vi "Grouped Interface.vi"() -> ()   [LabVIEW 2020, in "Grouped Interface.lvlib"]
doc: "This template is based off of the Queued Message Handler design pattern and the Queued Message Handler project template that ships with LabVIEW.\n\nThe main difference is that the queue is private to this module and communication between modules is performed via Broadcast and Request events.\n\nRequest events are wrapped in public API methods and are handled in the Event Handling Loop (EHL) of this VI. Any module can register for Broadcast events sent by this module. The EHL generates messages based on user interface actions.\n\nThe Message Handling Loop (MHL) processes messages generated by the EHL, or by other messages. The messages are string values, so new messages can be added easily to the Message Cases case structure in the MHL. Each message cluster can also provide an optional value for Message Data, which is a variant that can be converted to whatever message-specific data is required.\n_____\nBased on DQMH Project Template 7.0.1.1316."
uses:
  Grouped Interface.lvlib
  Grouped Interface/User Data--cluster.ctl
  <vilib>/Utility/miscctls.llb/LVRectTypeDef.ctl
  <vilib>/Utility/miscctls.llb/LVPointTypeDef.ctl
  Grouped Interface/Window Size Change Arguments--cluster.ctl
  Grouped Interface/Item Selected Arguments--cluster.ctl
  b692cfee-ccc7-4fcf-b071-59a242409c2d.vi
  6dcf879b-e50e-4c79-86d4-cf94ad6efafd.vi
  83f7a507-39ed-4955-bda1-3ff58afc1cf6.vi
  e3bdbc03-a268-4972-8073-54fcde4bb4c7.vi
  aefe27f5-81e8-4736-98ba-c14e2c182a52.vi
  b14c7c30-2e35-4566-a836-13db9432b85a.vi
  <userlib>/_NEVSTOP/Communicable State Machine(CSM)/AdvanceAPI/CSM - Revert Arguments-Safe String.vi
  <userlib>/_NEVSTOP/Communicable State Machine(CSM)/_Shared/Trim Single-line Text.vi
  <userlib>/_NEVSTOP/Communicable State Machine(CSM)/AdvanceAPI/CSM - Make String Arguments Safe.vi
  <userlib>/_NEVSTOP/Communicable State Machine(CSM)/AdvanceAPI/CSM - Break Down Multiple States String.vi
  <userlib>/_NEVSTOP/Communicable State Machine(CSM)/AdvanceAPI/CSM - Compact Multiple States.vi
  <userlib>/_NEVSTOP/Communicable State Machine(CSM)/AdvanceAPI/CSM - Keywords.vi
  <userlib>/_NEVSTOP/Communicable State Machine(CSM)/addons/API-String-Arugments-Support/_Support/Convert API String Arguments to Data(variant).vi
  <userlib>/_NEVSTOP/Communicable State Machine(CSM)/addons/API-String-Arugments-Support/_Support/Data To API String Arguments.vi
  <vilib>/Comparison/Equal/Equal Functor/Equal Functor.lvclass
  <userlib>/_NEVSTOP/Communicable State Machine(CSM)/Communicable State Machine.lvlib
panel:
  in  "min":bool
  in  "close":bool
  in  "Name (\"\" to Use UUID)":string="Main UI"
  out "State History":string
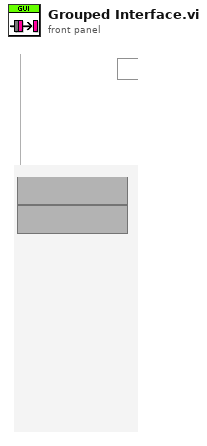
[diagram p1: front panel]
types:
  T1 = enum32{"Invalid", "Standard", "Closed", "Hidden", "Minimized", "Maximized"}
  T2 = enum32{"invalid app kind", "Development System", "Run Time System", "Student Edition", "Embedded LabVIEW", "Evaluation", "Custom"}
  T3 = typedef "Grouped Interface.lvlib/User Data--cluster.ctl" = cluster{"SubPanels":refnum<vi>[], "Interface Module List":string[], "Window Bounds":T4, "Function Module List":set{string}}
  T4 = typedef "LVRectTypeDef.ctl" = cluster{"Left":i16, "Top":i16, "Right":i16, "Bottom":i16}
  T5 = typedef "Grouped Interface.lvlib/Window Size Change Arguments--cluster.ctl" = cluster{"Module Name":string, "Window Size":T4}
  T6 = typedef "Grouped Interface.lvlib/Item Selected Arguments--cluster.ctl" = cluster{"Module Name":string, "Item Name":string}
  T7 = typedef "Communicable State Machine.lvlib/_CSM_Response Source Message.ctl" = cluster{"‘State":string, "’Arguments":string, "’Error":errorcluster}
  T8 = cluster{"Current VI Reference":refnum<vi>, "Close Panel on Exit?":bool}
  T9 = cluster{"Core":cluster{"Current VI Reference":refnum<vi>, "Close Panel on Exit?":bool}, "User Data":T3}
  T10 = typedef "LVPointTypeDef.ctl" = cluster{"Horizontal":i16, "Vertical":i16}
  T11 = typedef "Grouped Interface.lvlib/Module Definition--cluster.ctl" = cluster{"模块名称":string, "项定义":T12[]}
  T12 = typedef "Grouped Interface.lvlib/Function Item--cluster.ctl" = cluster{"项名":string, "符号图形路径":path}
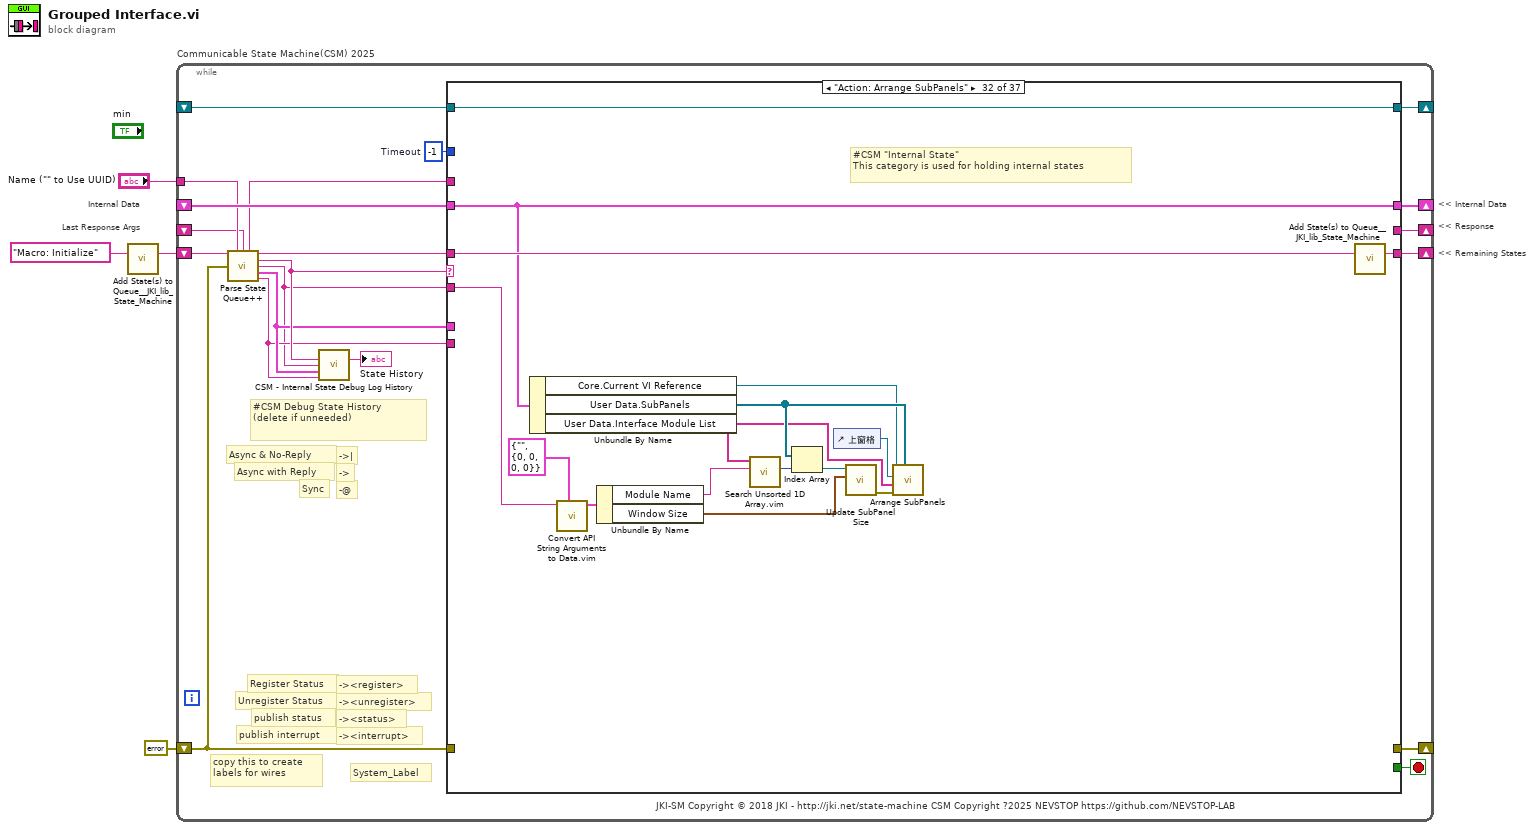
[diagram p0: block diagram]
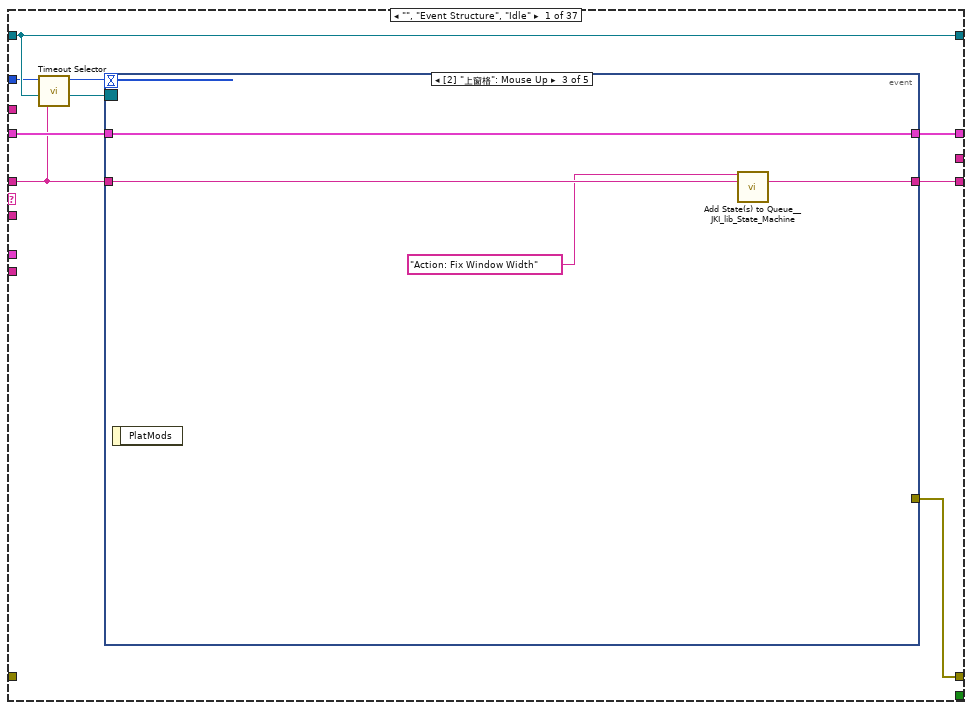
[diagram p2: hidden frame]
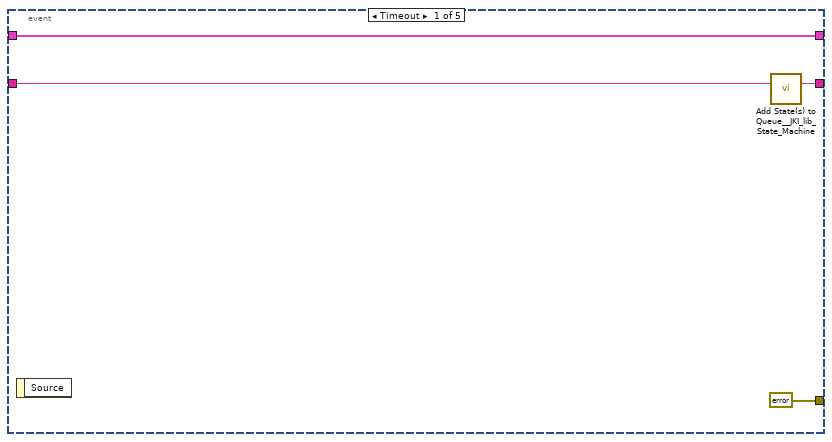
[diagram p3: hidden frame]
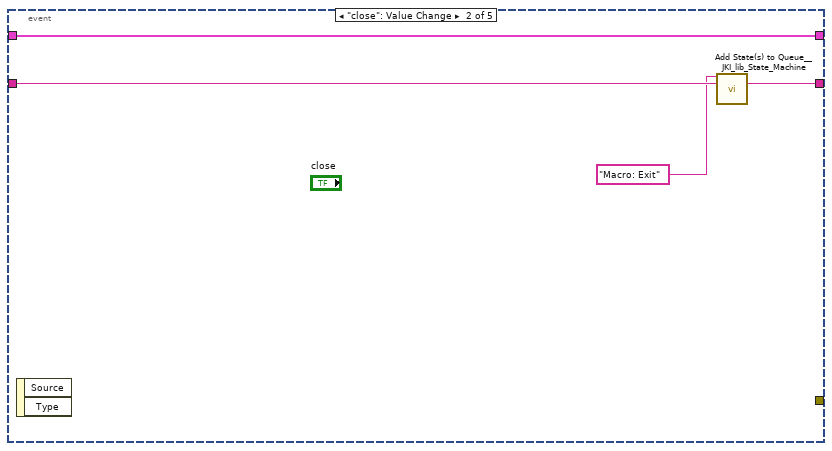
[diagram p4: hidden frame]
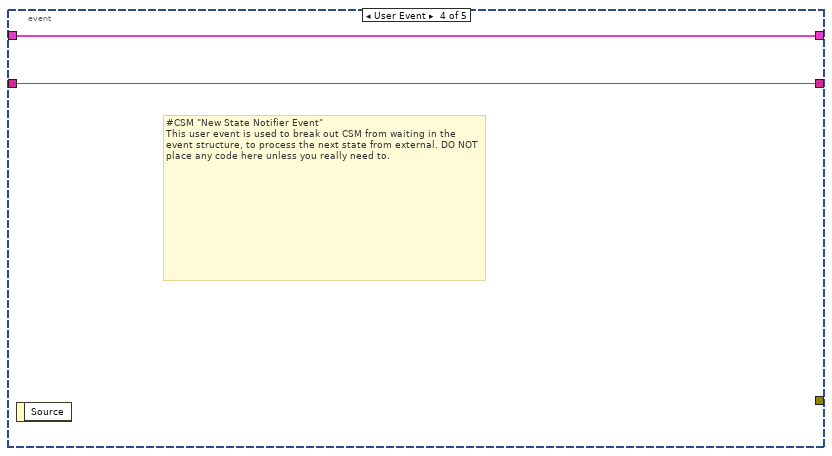
[diagram p5: hidden frame]
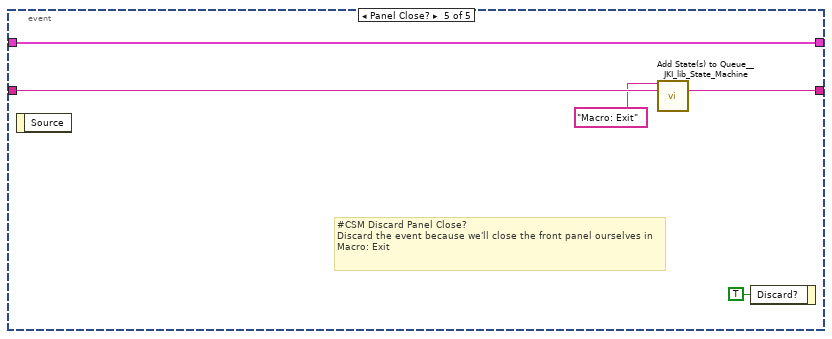
[diagram p6: hidden frame]
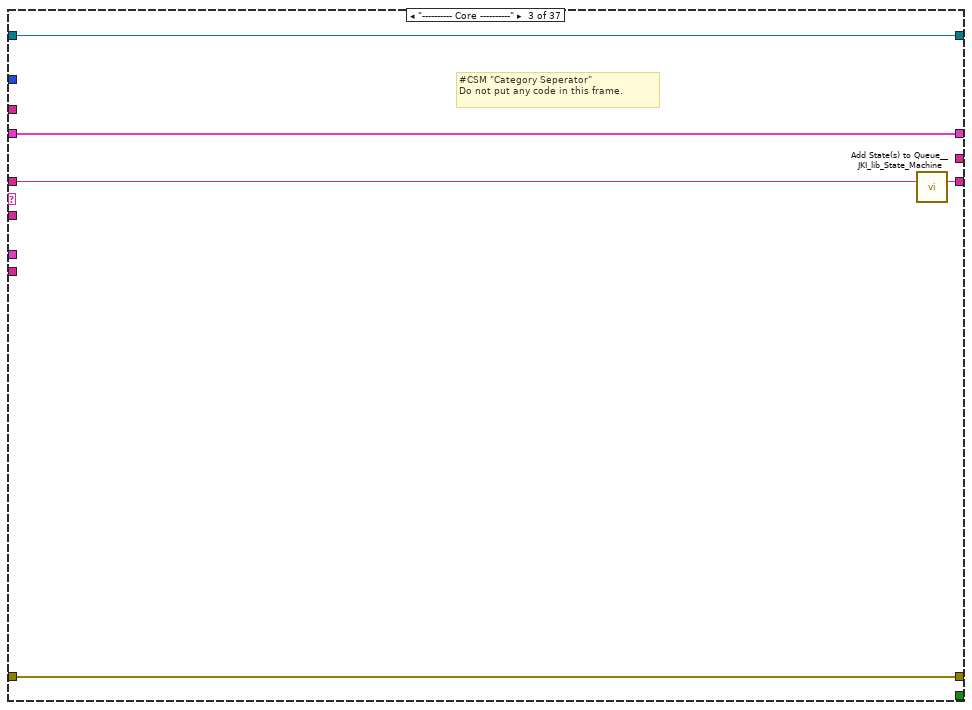
[diagram p8: hidden frame]
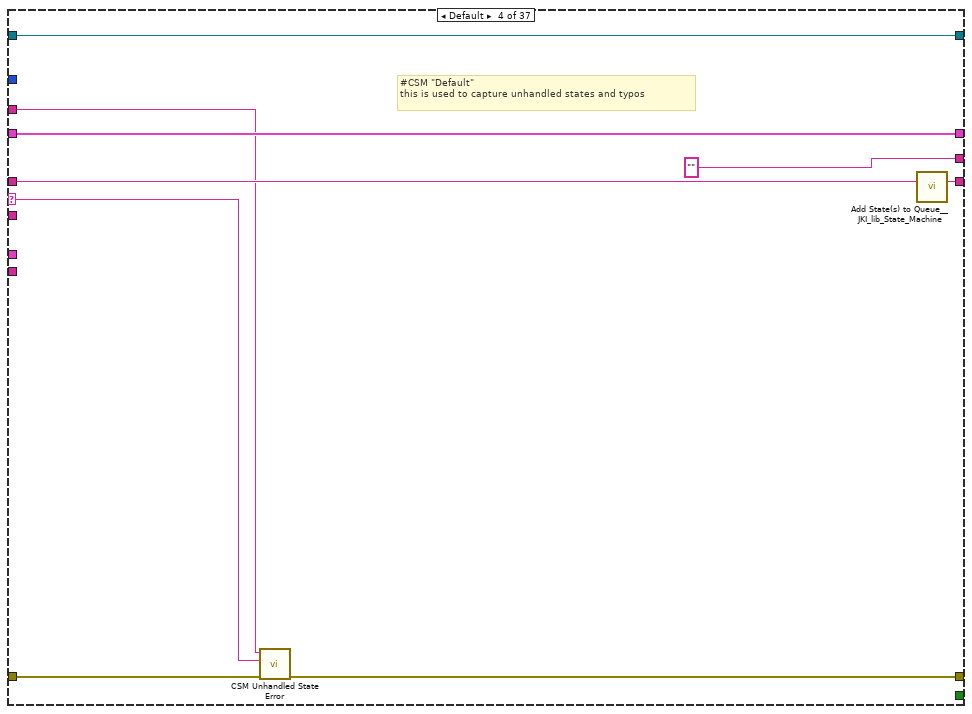
[diagram p9: hidden frame]
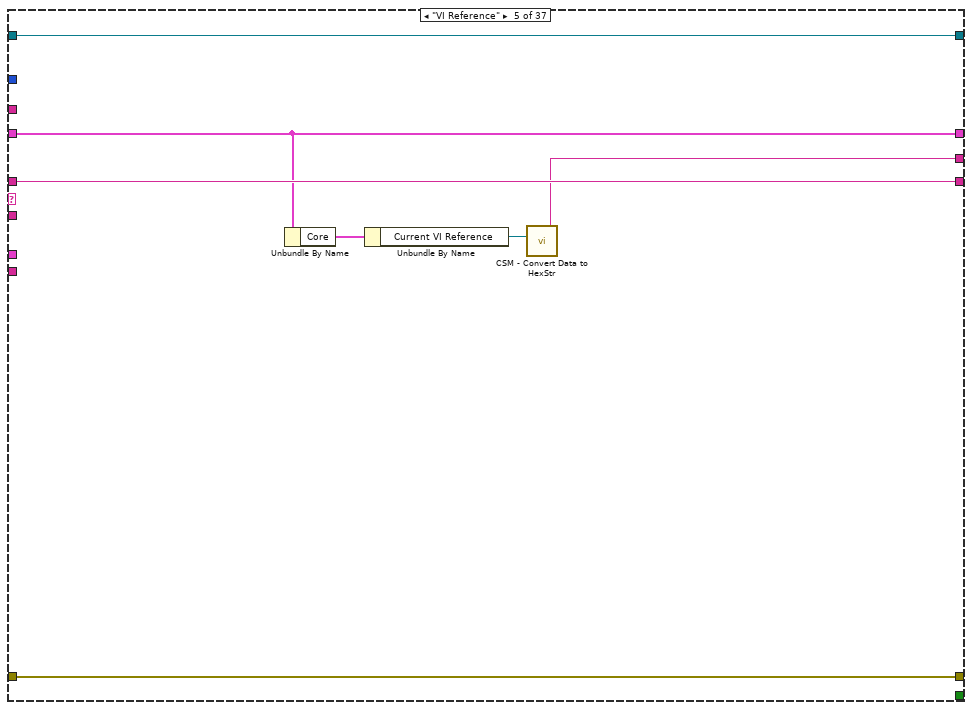
[diagram p10: hidden frame]
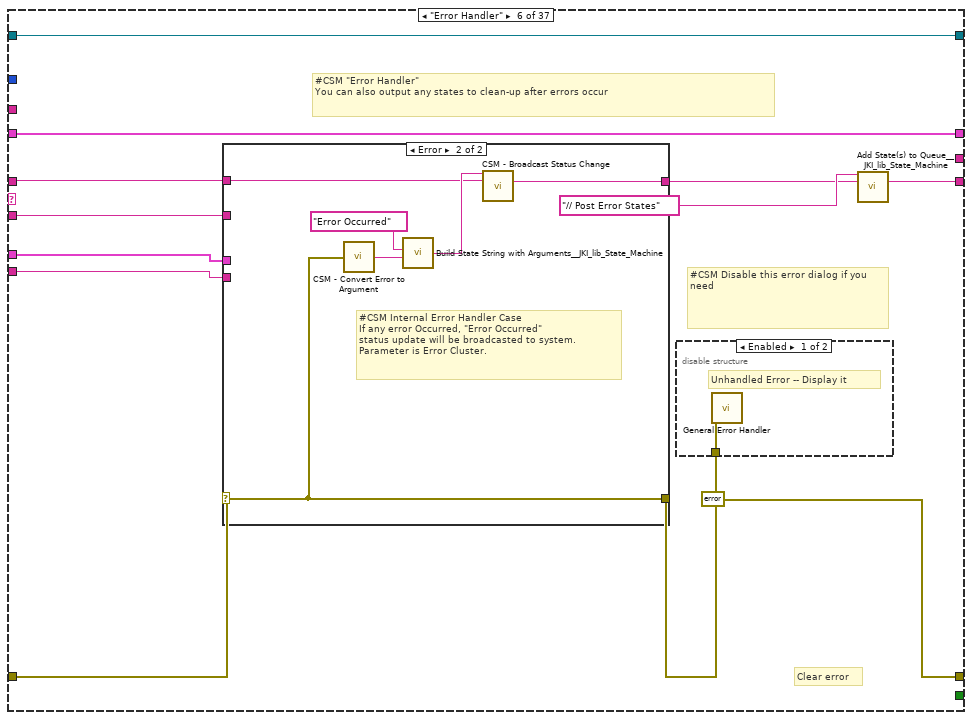
[diagram p11: hidden frame]
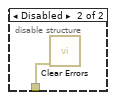
[diagram p12: hidden frame]
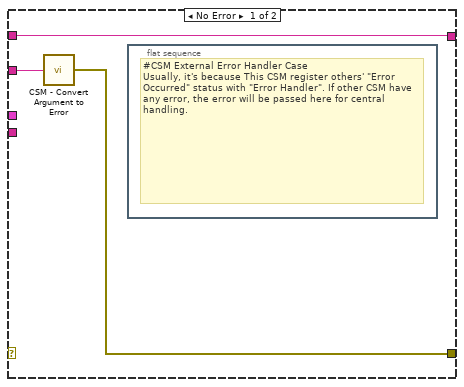
[diagram p13: hidden frame]
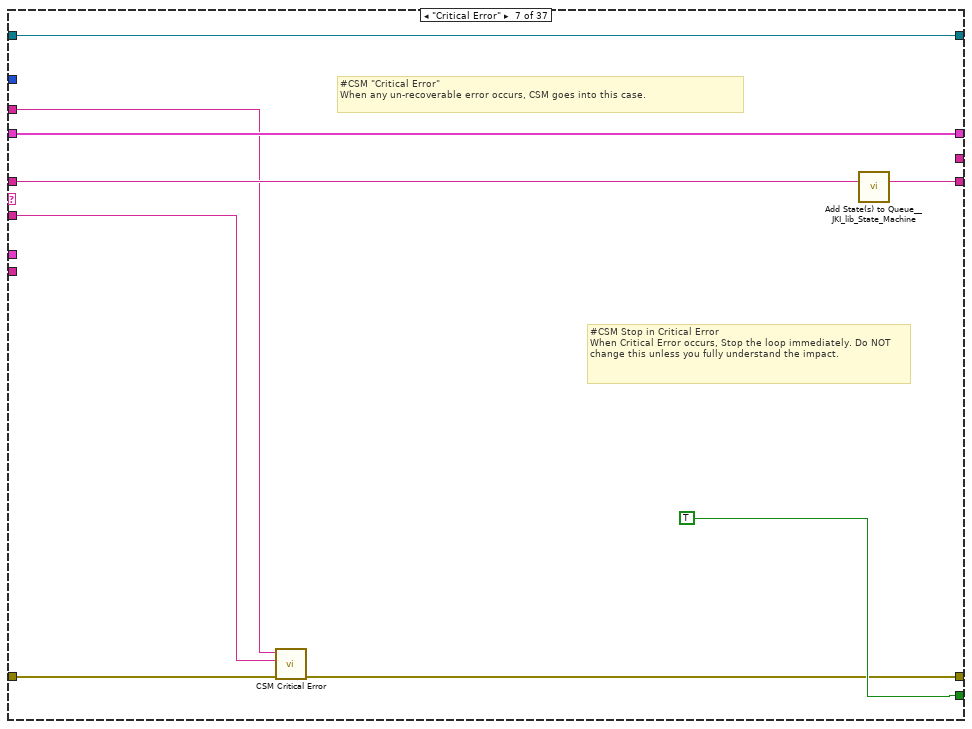
[diagram p14: hidden frame]
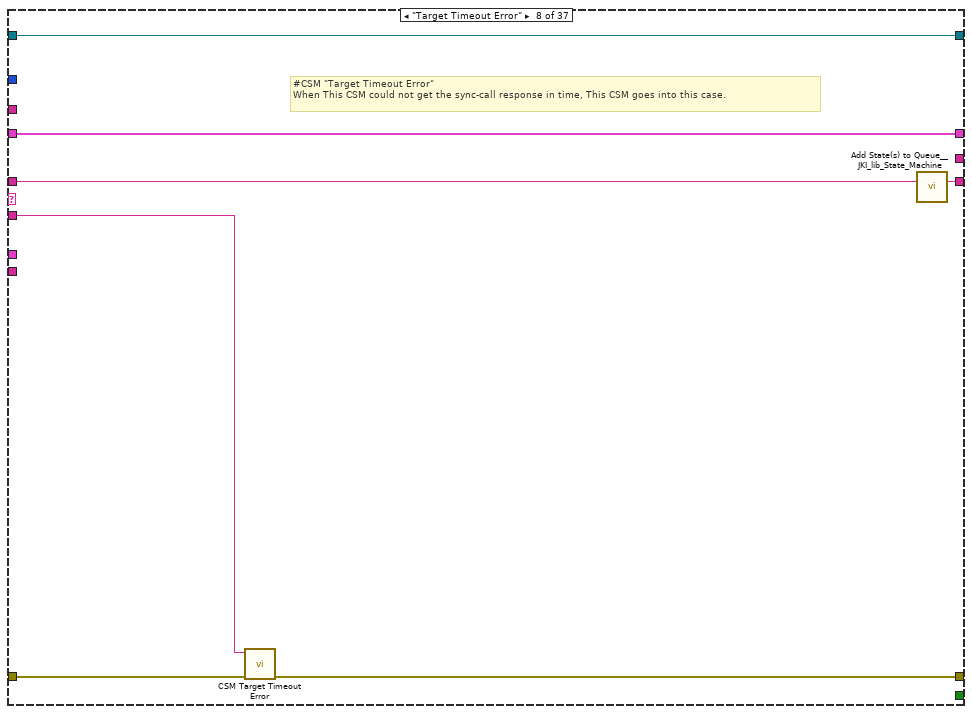
[diagram p15: hidden frame]
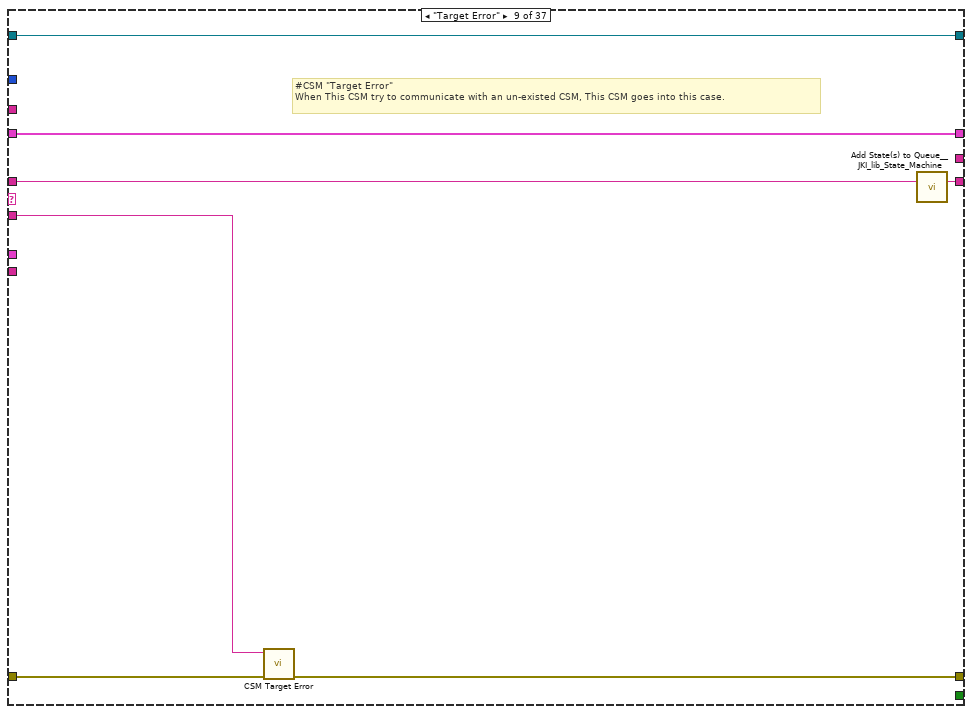
[diagram p16: hidden frame]
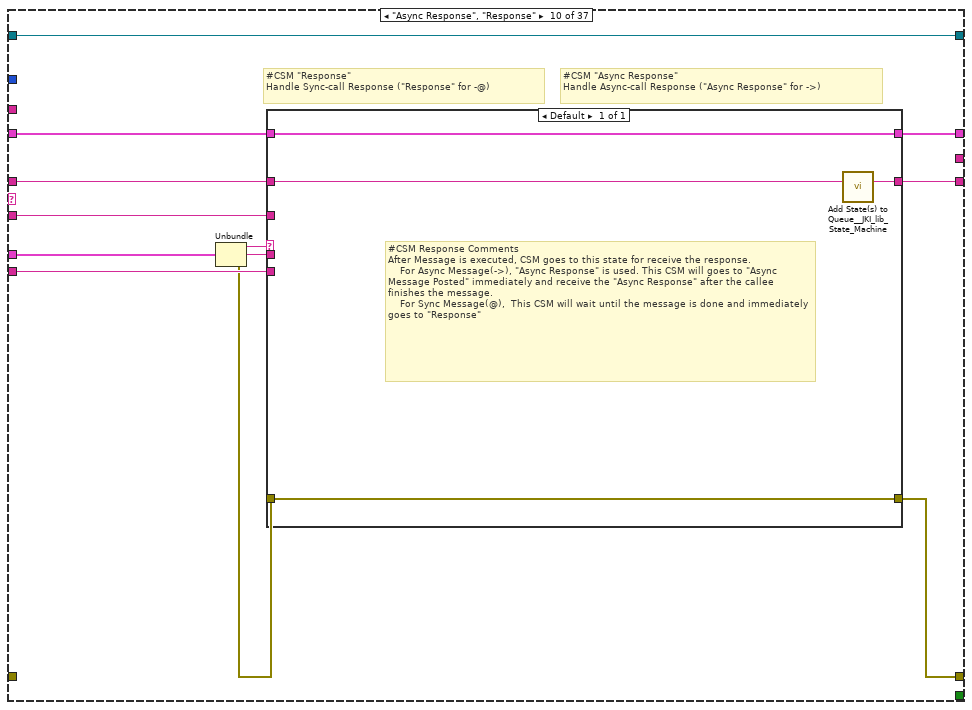
[diagram p17: hidden frame]
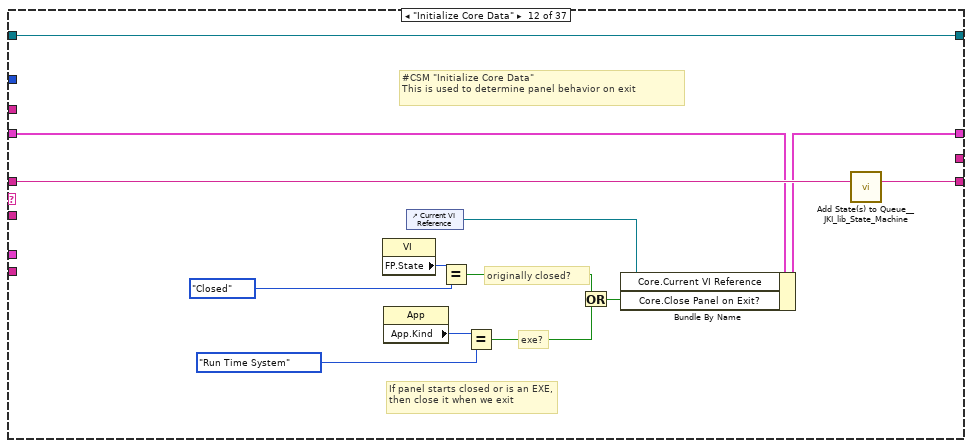
[diagram p19: hidden frame]
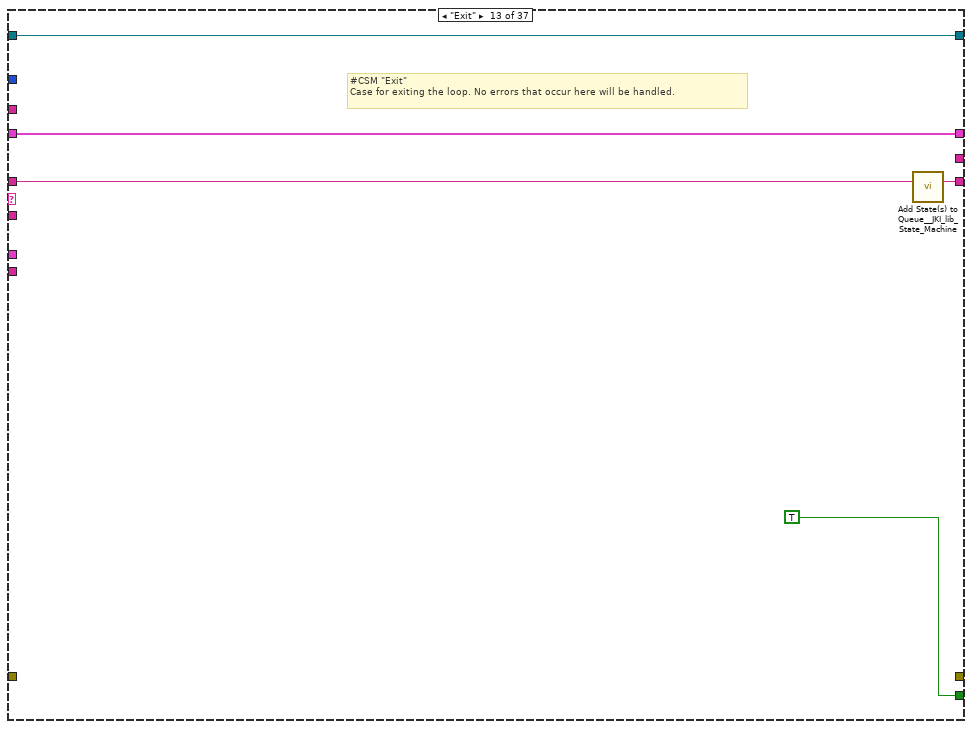
[diagram p20: hidden frame]
diagram:
  # "Last Response Args"
  # "Internal Data"
  # "<< Internal Data"
  # "<< Response"
  # "<< Remaining States"
  n1 = call <vilib>:"Add State(s) to Queue__JKI_lib_State_Machine.vi"("State(s) in (\"\")"="Macro: Initialize" ("Init State(\"Macro: Initialize\")")) -> ("States Out"=w1:string)  [unwired: 14 in]
  n2 = while "Communicable State Machine(CSM) 2025" {
    shift-right: [w19] -> _
    shift-left: _ -> [w18]
    shift-right: [w22] -> _
    shift-left: errorcluster {"status"=FALSE, "code"=0, "source"=""} ("error out") -> [w16]
    shift-right: [w21] -> _
    shift-left: w1 -> [w23]
    tunnel: "Name (\"\" to Use UUID)" -> [w12]
    shift-right: [w15] -> _
    shift-left: _ -> [w7]
    shift-right: [w14] -> _
    shift-left: _ -> [w13]
    stop <- w20 stop-if-true
    w17 = -1  # Timeout
    # "#CSM Debug State History\n(delete if unneeded)"
    # "-><interrupt>"
    # "-><status>"
    # "-><unregister>"
    # "-><register>"
    # "-@"
    # "->"
    # "->|"
    # "publish interrupt"
    # "publish status"
    # "Unregister Status"
    # "Register Status"
    # "Sync"
    # "Async with Reply"
    # "Async & No-Reply"
    # "copy this to create labels for wires"
    # "System_Label"
    # "JKI-SM Copyright © 2018 JKI - http://jki.net/state-machine CSM Copyright ?2025 NEVSTOP https://github.com/NEVSTOP-LAB"
    n3 = call <userlib>:"Parse State Queue++.vi"("State Queue"=w23, "Name (\"\" to Use UUID)"=w12, "Response Arguments"=w7, "Previous Error"=w16) -> ("Name Used"=w8:string, "Remaining States"=w24:string, "Current State"=w11:string, "Arguments"=w6:string, "Additional Information"=w10:T7, "Source CSM"=w9:string)  [unwired: 6 in]
    n4 = call <userlib>:"CSM - Internal State Debug Log History.vi"("State"=w11, "Arguments (\"\")"=w6, ">> Response Source Message >>"=w10, "Source (\"\")"=w9) -> ("Debug Log"=→"State History":string)  [unwired: 11 in]
    n5 = case shown="\"Action: Arrange SubPanels\"" w11 {
      selector: w11 -> [_ _ _ w62 _ _ _ _ _ _ _ _ _ _ _ _ _ _ _ _ _ _ _ _ _ _ _ _ _ _ _ _ _ _ _ _ _]
      tunnel: w24 -> [w25 w54 w59 w68 w74 w80 w106 w114 w121 w131 w140 w153 w158 w162 w181 w187 w191 w198 w202 w206 w223 w229 w240 w304 w309 w320 w323 w327 w334 w341 w352 w371 w376 w408 w429 w442 w452]
      tunnel: w6 -> [_ _ _ _ _ w78 w102 w109 w117 w125 _ _ _ _ _ _ _ _ _ _ _ w225 w235 _ _ _ _ w325 w332 _ _ w368 w381 _ _ w439 w448]
      tunnel: w18 -> [w31 w53 w56 w66 w73 w86 w107 w112 w119 w129 w139 w147 w156 w160 _ w183 w189 w197 w201 w204 w221 w227 w237 w302 w307 w318 w322 w330 w337 w339 w347 w365 w378 w394 w423 w437 w447]
      tunnel: [w30 _ w57 w60 w75 errorcluster {"status"=FALSE, "code"=0, "source"=""} ("error out") w99 w108 w115 w128 _ _ _ _ _ w184 _ w192 w200 _ _ w226 w238 _ _ _ _ _ _ _ _ _ _ _ _ _ _] -> w22
      tunnel: w16 -> [_ _ w57 w61 w75 w84 w100 w110 w116 _ _ _ _ _ _ _ _ _ _ _ _ _ _ _ _ _ _ _ _ _ _ _ _ _ _ _ _]
      tunnel: [w32 w54 w58 w67 w74 w82 w105 w113 w120 w132 w140 w152 w157 w161 w180 w186 w190 w198 w202 w205 w222 w228 w239 w303 w308 w319 w323 w328 w335 w340 w351 w370 w375 w407 w428 w441 w451] -> w21
      tunnel: [_ _ _ _ _ _ TRUE _ _ _ _ _ TRUE _ _ _ _ _ _ _ _ _ _ _ _ _ _ _ _ _ _ _ _ _ _ _ _] -> w20
      tunnel: [w29 w53 w56 w66 w73 w86 w107 w112 w119 w130 w139 w151 w156 w160 w179 w183 w189 w197 w201 w204 w221 w227 w237 w302 w307 w318 w322 w330 w337 w339 w345 w365 w377 w394 w423 w436 w444] -> w19
      tunnel: w17 -> [w27 _ _ _ _ _ _ _ _ _ _ _ _ _ _ _ _ _ _ _ _ _ _ _ _ _ _ _ _ _ _ _ _ _ _ _ _]
      tunnel: w9 -> [_ _ _ _ _ w77 _ _ _ w126 _ _ _ _ _ _ _ _ _ _ _ _ _ _ _ _ _ _ _ _ _ _ _ _ _ _ _]
      tunnel: w10 -> [_ _ _ _ _ w76 _ _ _ w127 _ _ _ _ _ _ _ _ _ _ _ _ _ _ _ _ _ _ _ _ _ _ _ _ _ _ _]
      tunnel: [_ _ _ "" w69 _ _ _ _ _ _ _ _ _ _ _ _ _ _ _ _ _ _ _ _ _ _ _ _ _ _ _ _ _ _ _ _] -> w15
      tunnel: [w28 w52 w55 w64 w72 w85 w103 w111 w118 w133 w138 w141 w154 w159 w177 w182 w188 w196 w199 w203 w220 w224 w234 w301 w305 w311 w321 w329 w336 w338 w350 w369 w382 w406 w427 w440 w450] -> w14
      tunnel: w13 -> [w28 w52 w55 w64 w72 w85 w103 w111 w118 w133 w138 w141 w154 w159 w177 w182 w188 _ w199 w203 w220 w224 w234 w301 w305 w311 w321 w329 w336 w338 w350 w369 w382 w406 w427 w440 w450]
      tunnel: w8 -> [_ _ _ w63 _ _ w101 _ _ _ _ _ _ _ _ _ _ w195 _ _ w214 _ _ _ _ _ _ _ _ _ _ _ _ w404 _ _ _]
      frame "", "Event Structure", "Idle" {
        n6 = call <userlib>:"Timeout Selector.vi"("Remaining States"=w25, "Timeout Expected"=w27) -> ("Timeout"=w26:i32)  [unwired: 5 in]
        n7 = event shown="[2] \"上窗格\": Mouse Up" {
          selector: w28 -> [_ _ _ _ _]
          dyn-events: _ -> [_ _ _ _ _]
          timeout: w26 -> [_ _ _ _ _]
          tunnel: w25 -> [w36 w38 w42 w45 w51]
          tunnel: [w35 w39 w43 w45 w50] -> w32
          tunnel: w31 -> [w34 w40 w44 w46 w49]
          tunnel: [errorcluster {"status"=FALSE, "code"=0, "source"=""} ("error out") _ _ _ _] -> w30
          tunnel: [w34 w40 w44 w46 w49] -> w29
          event Timeout {
            n8 = event-data() -> ()  [unwired: 1 in, 1 out]
            n9 = call <vilib>:"Add State(s) to Queue__JKI_lib_State_Machine.vi"("State(s) in (\"\")"=w36) -> ("States Out"=w35:string)  [unwired: 14 in]
          }
          event "close": Value Change {
            n10 = event-data() -> ()  [unwired: 1 in, 2 out]
            n11 = call <vilib>:"Add State(s) to Queue__JKI_lib_State_Machine.vi"("State(s) in Front (\"\")"="Macro: Exit" ("State(s) in Front (\"\")"), "State(s) in (\"\")"=w38) -> ("States Out"=w39:string)  [unwired: 13 in]
          }
          event Mouse Up {
            n12 = event-data() -> ()  [unwired: 1 in, 1 out]
            n13 = call <vilib>:"Add State(s) to Queue__JKI_lib_State_Machine.vi"("State(s) in Front (\"\")"="Action: Fix Window Width" ("State(s) in Front (\"\")"), "State(s) in (\"\")"=w42) -> ("States Out"=w43:string)  [unwired: 13 in]
          }
          event User Event {
            # "#CSM \"New State Notifier Event\"\nThis user event is used to break out CSM from waiting in the event structure, to process the next state from external. DO NOT place any code here unless you really need to."
            n14 = event-data() -> ()  [unwired: 1 in, 1 out]
          }
          event Panel Close? {
            # "#CSM Discard Panel Close?\nDiscard the event because we'll close the front panel ourselves in Macro: Exit"
            n15 = event-data() -> ()  [unwired: 1 in, 1 out]
            n16 = call <vilib>:"Add State(s) to Queue__JKI_lib_State_Machine.vi"("State(s) in Front (\"\")"="Macro: Exit", "State(s) in (\"\")"=w51) -> ("States Out"=w50:string)  [unwired: 13 in]
            n17 = event-data("Discard?"=TRUE) -> ()  [unwired: 1 in, 1 out]
          }
        }
      }
      frame "CSM Documentation" {
        # "#CSM State Syntax\n\n// Comment line, all text to the right of “//” will be ignored\n// Local Message Example\nDoSth: DoA >> Arguments\n\n// Sync Call Example\nAPI: xxxx >> Arguments -@ TargetModule\n\n// Async Call Example\nAPI: xxxx >> Arguments -> TargetModule\n\n// Async Call without Reply Example\nAPI: xxxx >> Arguments ->| TargetModule\n\n// Broadcast normal status:\nStatus >> StatusArguments  -><status>\n\n// Broadcast Interrupt status:\nInterrupt >> StatusArguments  -><interrupt>\n\n// Register Source Module's status to Handler Module\nStatus@Source Module >> Handler Module@Handler Module -><register>\n\n// Unegister Source Module's status\nStatus@Source Module >> Handler Module -><unregister>"
        # "#CSM README FIRST\n\nCommunicable State Machine(CSM) is a LabVIEW application framework that builds upon JKI State Machine(JKISM). It follows the pattern of JKISM and extends the keywords to describe message communication between modules, including concepts such as Sync-Message, Async-Message, Subscription/Unsubscription of status - essential elements for creating reusable code modules. For more information, please visit the CSM wiki: https://nevstop-lab.github.io/CSM-Wiki/\n\nFor instructions on JKI State Machine, visit: \n    http://jki.net/state-machine/\nFor information about CSM, visit: \n    https://github.com/NEVSTOP-LAB"
        # "#CSM \"Documentation\"\nCase for holding CSM Documenation"
      }
      frame "---------- Core ----------" {
        # "#CSM \"Category Seperator\"\nDo not put any code in this frame."
        n18 = call <vilib>:"Add State(s) to Queue__JKI_lib_State_Machine.vi"("State(s) in (\"\")"=w59) -> ("States Out"=w58:string)  [unwired: 14 in]
      }
      frame Default {
        # "#CSM \"Default\"\nthis is used to capture unhandled states and typos"
        n19 = call <userlib>:"CSM Unhandled State Error.vi"("error in (no error)"=w61, "Undefined State"=w62, "CSM Name"=w63) -> ("error out"=w60:errorcluster)  [unwired: 8 in]
        n20 = call <vilib>:"Add State(s) to Queue__JKI_lib_State_Machine.vi"("State(s) in (\"\")"=w68) -> ("States Out"=w67:string)  [unwired: 14 in]
      }
      frame "VI Reference" {
        n21 = Unbundle By Name(w73) -> ("Core"=w71:T8)
        n22 = Unbundle By Name(w71) -> ("Current VI Reference"=w70:refnum<vi>)
        n23 = call <userlib>:"CSM - Convert Data to HexStr.vi"("Variant"=w70) -> ("HEX String (0-9,A-F)"=w69:string)  [unwired: 8 in]
      }
      frame "Error Handler" {
        # "#CSM Disable this error dialog if you need"
        # "#CSM \"Error Handler\"\nYou can also output any states to clean-up after errors occur"
        # "Clear error"
        n24 = case shown="Error" w84 {
          selector: w84 -> [_ w93]
          tunnel: [w91 w95] -> w81
          tunnel: w80 -> [w91 w94]
          tunnel: [w90 w93] -> w79
          tunnel: w78 -> [w92 _]
          tunnel: w77 -> [_ _]
          tunnel: w76 -> [_ _]
          frame No Error {
            n25 = call <userlib>:"CSM - Convert Argument to Error.vi"("Argument"=w92) -> ("Error"=w90:errorcluster)  [unwired: 4 in]
            n26 = flat-sequence {
              frame #0 {
                # "#CSM External Error Handler Case\nUsually, it's because This CSM register others' \"Error Occurred\" status with \"Error Handler\". If other CSM have any error, the error will be passed here for central handling."
              }
            }
          }
          frame Error {
            # "#CSM Internal Error Handler Case \nIf any error Occurred, \"Error Occurred\" \nstatus update will be broadcasted to system.\nParameter is Error Cluster."
            n27 = call <userlib>:"CSM - Convert Error to Argument.vi"("Error"=w93) -> ("Argument"=w97:string)  [unwired: 4 in]
            n28 = call <vilib>:"Build State String with Arguments__JKI_lib_State_Machine.vi"("Arguments (\"\")"=w97, "State"="Error Occurred" ("Status with Arguments")) -> ("State with Arguments"=w96:string)  [unwired: 4 in]
            n29 = call <userlib>:"CSM - Broadcast Status Change.vi"("Status With Arguments"=w96, "State Queue"=w94) -> ("Remaining States"=w95:string)  [unwired: 13 in]
          }
        }
        n30 = disable-structure shown="Enabled" {
          disable-tunnel: w79 -> [w88 w89]
          frame Enabled {
            # "Unhandled Error -- Display it"
            n31 = call <vilib>:"General Error Handler.vi"("error in (no error)"=w88) -> ()  [unwired: 10 in, 5 out]
          }
          frame Disabled {
            n32 = call <vilib>:"Clear Errors.vi"("error in (no error)"=w89) -> ()  [unwired: 5 in, 2 out]
          }
        }
        n33 = call <vilib>:"Add State(s) to Queue__JKI_lib_State_Machine.vi"("State(s) in Front (\"\")"="// Post Error States", "State(s) in (\"\")"=w81) -> ("States Out"=w82:string)  [unwired: 13 in]
      }
      frame "Critical Error" {
        # "#CSM \"Critical Error\"\nWhen any un-recoverable error occurs, CSM goes into this case."
        # "#CSM Stop in Critical Error\nWhen Critical Error occurs, Stop the loop immediately. Do NOT change this unless you fully understand the impact."
        n34 = call <userlib>:"CSM Critical Error.vi"("error in (no error)"=w100, "Arugments (As Reason)"=w102, "CSM Name"=w101) -> ("error out"=w99:errorcluster)  [unwired: 8 in]
        n35 = call <vilib>:"Add State(s) to Queue__JKI_lib_State_Machine.vi"("State(s) in (\"\")"=w106) -> ("States Out"=w105:string)  [unwired: 14 in]
      }
      frame "Target Timeout Error" {
        # "#CSM \"Target Timeout Error\"\nWhen This CSM could not get the sync-call response in time, This CSM goes into this case."
        n36 = call <userlib>:"CSM Target Timeout Error.vi"("error in (no error)"=w110, "Arguments (As CSM Name)"=w109) -> ("error out"=w108:errorcluster)  [unwired: 9 in]
        n37 = call <vilib>:"Add State(s) to Queue__JKI_lib_State_Machine.vi"("State(s) in (\"\")"=w114) -> ("States Out"=w113:string)  [unwired: 14 in]
      }
      frame "Target Error" {
        # "#CSM \"Target Error\"\nWhen This CSM try to communicate with an un-existed CSM, This CSM goes into this case."
        n38 = call <userlib>:"CSM Target Error.vi"("error in (no error)"=w116, "Arguments (As CSM Name)"=w117) -> ("error out"=w115:errorcluster)  [unwired: 9 in]
        n39 = call <vilib>:"Add State(s) to Queue__JKI_lib_State_Machine.vi"("State(s) in (\"\")"=w121) -> ("States Out"=w120:string)  [unwired: 14 in]
      }
      frame "Async Response", "Response" {
        # "#CSM \"Async Response\"\nHandle Async-call Response (\"Async Response\" for ->)"
        # "#CSM \"Response\"\nHandle Sync-call Response (\"Response\" for -@)"
        n40 = Unbundle(w127) -> ("‘State"=w124:string, "’Arguments"=w123:string, "’Error"=w122:errorcluster)
        n41 = case shown="Default" w124 {
          tunnel: [w134] -> w132
          tunnel: w131 -> [w135]
          tunnel: [w137] -> w130
          tunnel: w129 -> [w137]
          tunnel: [w136] -> w128
          tunnel: w122 -> [w136]
          tunnel: w126 -> [_]
          tunnel: w125 -> [_]
          tunnel: w123 -> [_]
          frame Default {
            # "#CSM Response Comments\nAfter Message is executed, CSM goes to this state for receive the response.\n    For Async Message(->), \"Async Response\" is used. This CSM will goes to \"Async Message Posted\" immediately and receive the \"Async Response\" after the callee finishes the message.\n    For Sync Message(@),  This CSM will wait until the message is done and immediately goes to \"Response\""
            n42 = call <vilib>:"Add State(s) to Queue__JKI_lib_State_Machine.vi"("State(s) in (\"\")"=w135) -> ("States Out"=w134:string)  [unwired: 14 in]
          }
        }
      }
      frame "Async Message Posted" {
        # "#CSM \"Async Message Posted\"\nAfter Async Message is posted (-> or ->| ), CSM goes to this state for post-action.\nYou can use Argument - State to tell which Async Message is called."
      }
      frame "Initialize Core Data" {
        # "#CSM \"Initialize Core Data\"\nThis is used to determine panel behavior on exit"
        # "originally closed?"
        # "exe?"
        # "If panel starts closed or is an EXE, then close it when we exit"
        n43 = property class="VI"() -> ("FP.State"=w144:T1)  [unwired: 2 in, 2 out]
        n44 = property class="App"() -> ("App.Kind"=w150:T2)  [unwired: 2 in, 2 out]
        n45 = control-ref of="Current VI Reference"() -> (w145:refnum<vi>)
        n46 = Equal?(x=w144, y=T1."Closed" ("Front Panel Window:State")) -> (x = y?=w142:bool)
        n47 = Equal?(x=w150, y=T2."Run Time System" ("Application:Kind")) -> (x = y?=w148:bool)
        n48 = Or(x=w142, y=w148) -> (x .or. y?=w146:bool)
        n49 = Bundle By Name(cluster=w147, "Core.Current VI Reference"=w145, "Core.Close Panel on Exit?"=w146) -> (w151:T9)
        n50 = call <vilib>:"Add State(s) to Queue__JKI_lib_State_Machine.vi"("State(s) in (\"\")"=w153) -> ("States Out"=w152:string)  [unwired: 14 in]
      }
      frame "Exit" {
        # "#CSM \"Exit\"\nCase for exiting the loop. No errors that occur here will be handled."
        n51 = call <vilib>:"Add State(s) to Queue__JKI_lib_State_Machine.vi"("State(s) in (\"\")"=w158) -> ("States Out"=w157:string)  [unwired: 14 in]
      }
      frame "---------- Data ----------" {
        # "#CSM \"Category Seperator\"\nDo not put any code in this frame."
        n52 = call <vilib>:"Add State(s) to Queue__JKI_lib_State_Machine.vi"("State(s) in (\"\")"=w162) -> ("States Out"=w161:string)  [unwired: 14 in]
      }
      frame "Data: Initialize" {
        w178 = T8 {"Current VI Reference"=refnum, "Close Panel on Exit?"=FALSE}  # Core
        # "#CSM  do not delete - used by framework"
        # "#CSM Data names and types of shift register data are defined by this bundle."
        # "#CSM \"Data: Initialize\"\nInitialize the shift-register data, here.\n(data names are defined by what you wire into the bundle function)"
        n53 = control-ref of="M1"() -> (w169:refnum<vi>)
        n54 = control-ref of="M2"() -> (w170:refnum<vi>)
        n55 = control-ref of="M3"() -> (w171:refnum<vi>)
        n56 = control-ref of="M4"() -> (w166:refnum<vi>)
        n57 = control-ref of="M5"() -> (w167:refnum<vi>)
        n58 = control-ref of="M6"() -> (w168:refnum<vi>)
        n59 = control-ref of="M7"() -> (w172:refnum<vi>)
        n60 = control-ref of="M8"() -> (w173:refnum<vi>)
        n61 = control-ref of="M9"() -> (w174:refnum<vi>)
        n62 = control-ref of="M10"() -> (w175:refnum<vi>)
        n63 = Build Array(w169, w170, w171, w166, w167, w168, w172, w173, w174, w175) -> (w165:refnum<vi>[])
        n64 = property class="VI"() -> ("Front Panel.WinBounds"=w163:T4)  [unwired: 2 in, 2 out]
        n65 = Bundle By Name(cluster=T3 {"SubPanels"=[], "Interface Module List"=[], "Window Bounds"={"Left"=0, "Top"=0, "Right"=0, "Bottom"=0}, "Function Module List"={}} ("User Data"), "SubPanels"=w165, "Window Bounds"=w163) -> (w164:T3)
        n66 = Bundle("Core"=w178, "User Data"=w164) -> (w179:T9)  [unwired: 1 in]
        n67 = call <vilib>:"Add State(s) to Queue__JKI_lib_State_Machine.vi"("State(s) in (\"\")"=w181) -> ("States Out"=w180:string)  [unwired: 14 in]
      }
      frame "Data: Cleanup" {
        # "#CSM \"Data: Cleanup\"\nCleanup any data and references, here.\n(this is called automatically, by the Macro: Exit)"
        n68 = Unbundle By Name(w183) -> ("Core.Current VI Reference"=w185:refnum<vi>)
        n69 = Close Reference(reference=w185) -> (error out=w184:errorcluster)  [unwired: 1 in]
        n70 = call <vilib>:"Add State(s) to Queue__JKI_lib_State_Machine.vi"("State(s) in (\"\")"=w187) -> ("States Out"=w186:string)  [unwired: 14 in]
      }
      frame "---------- Events ----------" {
        # "#CSM \"Category Seperator\"\nDo not put any code in this frame."
        n71 = call <vilib>:"Add State(s) to Queue__JKI_lib_State_Machine.vi"("State(s) in (\"\")"=w191) -> ("States Out"=w190:string)  [unwired: 14 in]
      }
      frame "Events: Register" {
        # "#CSM \"Events: Register\"\nRegister user event. New Message Event is registered to break CSM waiting in event structure by default."
        # "#CSM Register New Message Event\nRegister message event to break Waiting in Event structure."
        n72 = call <userlib>:"CSM - Get New State Notifier Event.vi"("Name (\"\" to Use UUID)"=w195) -> ("error out"=w193:errorcluster, "New State Notifier Event"=w194:refnum<user-event>)  [unwired: 9 in]
        n73 = register-events(error in=w193, w194) -> (reference out=w196:refnum<event-registration>, error out=w192:errorcluster)  [unwired: 1 in]
      }
      frame "Events: Unregister" {
        # "#CSM \"Events: Unregister\"\nUnregister user event."
        n74 = Unregister For Events(event registration refnum=w199) -> (error out=w200:errorcluster)  [unwired: 1 in]
      }
      frame "---------- UI ----------" {
        # "#CSM \"Category Seperator\"\nDo not put any code in this frame."
        n75 = call <vilib>:"Add State(s) to Queue__JKI_lib_State_Machine.vi"("State(s) in (\"\")"=w206) -> ("States Out"=w205:string)  [unwired: 14 in]
      }
      frame "UI: Initialize" {
        w218 = T10 {"Horizontal"=0, "Vertical"=0} ("Origin")
        # "#CSM \"UI: Initialize\"\nInitialize the User Interface, here.\n(this is called automatically, by the Macro: Init)"
        n76 = control-ref of="上窗格"() -> (w216:refnum<vi>)
        n77 = control-ref of="下窗格"() -> (w219:refnum<vi>)
        n78 = call "FramelessFP Drop-In.vi"("Pane in"=w216) -> ("error out"=w215:errorcluster)  [unwired: 10 in]
        n79 = property class="Pane"(reference=w216, "Origin"=w218) -> ()  [unwired: 1 in, 2 out]
        n80 = property class="Pane"(reference=w219, "PaneColor"=u32 16053492 ("Pane Color"), "Origin"=w218) -> ()  [unwired: 1 in, 2 out]
        n81 = call <vilib>:"Clear Errors.vi"("error in (no error)"=w215) -> ()  [unwired: 5 in, 2 out]
        n82 = call <userlib>:"CSM - Register Broadcast.vi"("CSM Name(Empty for Broadcast Event)"=w214, "Trigger"="Window Size Changed", "API (If \"\", Same as Trigger)"="Action: Arrange SubPanels" ("API (If \"\", Same as Trigger)")) -> ("CSM Name (Dup)"=w210:string, "error out"=w211:errorcluster)  [unwired: 11 in]
        n83 = call <userlib>:"CSM - Register Broadcast.vi"("CSM Name(Empty for Broadcast Event)"=w210, "Trigger"="Item Selected", "API (If \"\", Same as Trigger)"="Action: Launch Function" ("API (If \"\", Same as Trigger)"), "Error In"=w211) -> ()  [unwired: 10 in, 2 out]
        n84 = call <vilib>:"Add State(s) to Queue__JKI_lib_State_Machine.vi"("State(s) in (\"\")"=w223, "State(s) at Back (\"\")"="Action: Load Modules" ("API (If \"\", Same as Trigger)")) -> ("States Out"=w222:string)  [unwired: 13 in]
      }
      frame "UI: Cursor Set" {
        # "Argument"
        # "#CSM \"UI: Cursor Set\"\nSet and Unset Cursor Busy.\n(Usage: \"UI: Cursor Set >> Busy|Idle\")"
        n85 = disable-structure shown="TARGET_TYPE!=Windows" {
          disable-tunnel: [w231 _] -> w226
          disable-tunnel: w225 -> [w230 _]
          frame condition #0 (active) {
            n86 = case shown="\"Idle\", Default" w230 {
              tunnel: [w232 w233] -> w231
              frame "Idle", Default {
                n87 = call <vilib>:"Unset Busy.vi"() -> ("error out"=w232:errorcluster)  [unwired: 11 in]
              }
              frame "Busy" {
                n88 = call <vilib>:"Set Busy.vi"() -> ("error out"=w233:errorcluster)  [unwired: 10 in, 1 out]
              }
            }
          }
          frame condition #1 {
          }
        }
        n89 = call <vilib>:"Add State(s) to Queue__JKI_lib_State_Machine.vi"("State(s) in (\"\")"=w229) -> ("States Out"=w228:string)  [unwired: 14 in]
      }
      frame "UI: Front Panel State" {
        # "Argument"
        # "#CSM \"UI: Front Panel State\"\nSet Front Panel Open or Closed\n(Usage: \"UI: Front Panel State >> Open|Close\")"
        n90 = Unbundle By Name(w237) -> ("Core.Current VI Reference"=w236:refnum<vi>)
        n91 = case shown="\"Close\", \"Closed\"" w235 {
          tunnel: [w247 w260 w271 w283 w295] -> w238
          tunnel: w236 -> [w246 w258 w270 w282 w294]
          frame "Open", "Standard", Default {
            w241 = T1."Standard" ("State")
            n92 = property class="VI"(reference=w246) -> (reference out=w244:refnum<vi>, error out=w245:errorcluster, "FP.State"=w243:T1)  [unwired: 1 in]
            n93 = Not Equal?(x=w243, y=w241) -> (x != y?=w242:bool)
            n94 = case shown="True" w242 {
              tunnel: [w251 w253] -> w247
              tunnel: w245 -> [w250 w253]
              tunnel: w244 -> [w249 _]
              tunnel: w241 -> [w248 _]
              frame True {
                n95 = invoke class="VI" method="FP.Open"(reference=w249, error in=w250, "Activate"=TRUE, "State"=w248) -> (error out=w251:errorcluster)  [unwired: 1 in, 4 out]
              }
              frame False {
              }
            }
          }
          frame "Close", "Closed" {
            n96 = property class="VI"(reference=w258) -> (reference out=w257:refnum<vi>, error out=w259:errorcluster, "FP.State"=w255:T1)  [unwired: 1 in]
            n97 = Not Equal?(x=w255, y=T1."Closed" ("Front Panel Window:State")) -> (x != y?=w254:bool)
            n98 = case shown="True" w254 {
              tunnel: [w261 w264] -> w260
              tunnel: w259 -> [w261 w263]
              tunnel: w257 -> [_ w262]
              frame False {
              }
              frame True {
                n99 = invoke class="VI" method="FP.Close"(reference=w262, error in=w263) -> (error out=w264:errorcluster)  [unwired: 1 in, 2 out]
              }
            }
          }
          frame "Hidden", "Hide" {
            w265 = T1."Hidden" ("State")
            n100 = property class="VI"(reference=w270) -> (reference out=w268:refnum<vi>, error out=w269:errorcluster, "FP.State"=w267:T1)  [unwired: 1 in]
            n101 = Not Equal?(x=w267, y=w265) -> (x != y?=w266:bool)
            n102 = case shown="True" w266 {
              tunnel: [w275 w276] -> w271
              tunnel: w269 -> [w274 w276]
              tunnel: w268 -> [w273 _]
              tunnel: w265 -> [w272 _]
              frame True {
                n103 = invoke class="VI" method="FP.Open"(reference=w273, error in=w274, "State"=w272) -> (error out=w275:errorcluster)  [unwired: 2 in, 4 out]
              }
              frame False {
              }
            }
          }
          frame "Minimize", "Minimized" {
            w277 = T1."Minimized" ("State")
            n104 = property class="VI"(reference=w282) -> (reference out=w280:refnum<vi>, error out=w281:errorcluster, "FP.State"=w279:T1)  [unwired: 1 in]
            n105 = Not Equal?(x=w279, y=w277) -> (x != y?=w278:bool)
            n106 = case shown="False" w278 {
              tunnel: [w287 w288] -> w283
              tunnel: w281 -> [w286 w288]
              tunnel: w280 -> [w285 _]
              tunnel: w277 -> [w284 _]
              frame True {
                n107 = invoke class="VI" method="FP.Open"(reference=w285, error in=w286, "State"=w284) -> (error out=w287:errorcluster)  [unwired: 2 in, 4 out]
              }
              frame False {
              }
            }
          }
          frame "Maximize", "Maximized" {
            w289 = T1."Maximized" ("State")
            n108 = property class="VI"(reference=w294) -> (reference out=w292:refnum<vi>, error out=w293:errorcluster, "FP.State"=w291:T1)  [unwired: 1 in]
            n109 = Not Equal?(x=w291, y=w289) -> (x != y?=w290:bool)
            n110 = case shown="True" w290 {
              tunnel: [w299 w300] -> w295
              tunnel: w293 -> [w298 w300]
              tunnel: w292 -> [w297 _]
              tunnel: w289 -> [w296 _]
              frame True {
                n111 = invoke class="VI" method="FP.Open"(reference=w297, error in=w298, "State"=w296) -> (error out=w299:errorcluster)  [unwired: 2 in, 4 out]
              }
              frame False {
              }
            }
          }
        }
        n112 = call <vilib>:"Add State(s) to Queue__JKI_lib_State_Machine.vi"("State(s) in (\"\")"=w240) -> ("States Out"=w239:string)  [unwired: 14 in]
      }
      frame "---------- Macro ----------" {
        # "#CSM \"Category Seperator\"\nDo not put any code in this frame."
        n113 = call <vilib>:"Add State(s) to Queue__JKI_lib_State_Machine.vi"("State(s) in (\"\")"=w304) -> ("States Out"=w303:string)  [unwired: 14 in]
      }
      frame "Macro: Initialize" {
        w306 = "Data: Initialize\nInitialize Core Data\nEvents: Register\nUI: Initialize\nUI: Front Panel State >> Open"  # Data: Initialize Initialize Core Data Events: Register UI: Initialize UI: Front Panel State >> Open
        # "#CSM \"Macro: Initialize\"\nInitialization Macro (This is called once, when the VI starts)"
        n114 = call <vilib>:"Add State(s) to Queue__JKI_lib_State_Machine.vi"("State(s) in Front (\"\")"=w306, "State(s) in (\"\")"=w309) -> ("States Out"=w308:string)  [unwired: 13 in]
      }
      frame "Macro: Exit" {
        # "#CSM \"Macro: Exit\"\nExit Macro (This is called once, when the VI exits)"
        n115 = Unbundle By Name(w318) -> ("Core.Close Panel on Exit?"=w317:bool)
        n116 = Select(t="UI: Front Panel State >> Close", s=w317, f="") -> (s? t:f=w314:string)
        n117 = call <vilib>:"Add State(s) to Queue__JKI_lib_State_Machine.vi"("State(s) in Front (\"\")"="Action: Exit Modules ", "State(s) in (\"\")"=w314, "State(s) at Back (\"\")"="Data: Cleanup\nEvents: Unregister\nExit") -> ("States Out"=w312:string)  [unwired: 12 in]
        n118 = call <vilib>:"Add State(s) to Queue__JKI_lib_State_Machine.vi"("State(s) in Front (\"\")"=w312, "State(s) in (\"\")"=w320) -> ("States Out"=w319:string)  [unwired: 13 in]
      }
      frame "---------- API ----------" {
        # "#CSM \"Category Seperator\"\nDo not put any code in this frame."
      }
      frame "API: Unregister Window" {
        # "#CSM API Example\nCopy/Rename this case for your own API"
        n119 = call <vilib>:"Build State String with Arguments__JKI_lib_State_Machine.vi"("Arguments (\"\")"=w325, "State"="Action: Unregister Window") -> ("State with Arguments"=w324:string)  [unwired: 4 in]
        n120 = call <vilib>:"Add State(s) to Queue__jki_lib_state_machine.vi"("State(s) in Front (\"\")"=w324, "State(s) in (\"\")"=w327) -> ("States Out"=w328:string)  [unwired: 13 in]
      }
      frame "API: Register Window" {
        # "#CSM API Example\nCopy/Rename this case for your own API"
        n121 = call <vilib>:"Build State String with Arguments__JKI_lib_State_Machine.vi"("Arguments (\"\")"=w332, "State"="Action: Register Window") -> ("State with Arguments"=w331:string)  [unwired: 4 in]
        n122 = call <vilib>:"Add State(s) to Queue__jki_lib_state_machine.vi"("State(s) in Front (\"\")"=w331, "State(s) in (\"\")"=w334) -> ("States Out"=w335:string)  [unwired: 13 in]
      }
      frame "---------- Action ----------" {
        # "#CSM \"Category Seperator\"\nDo not put any code in this frame."
        n123 = call <vilib>:"Add State(s) to Queue__JKI_lib_State_Machine.vi"("State(s) in (\"\")"=w341) -> ("States Out"=w340:string)  [unwired: 14 in]
      }
      frame "Action: Load Modules" {
        # "#CSM \"Category Seperator\"\nDo not put any code in this frame."
        n124 = call <vilib>:"Application Directory.vi"() -> ("Application Directory"=w342:path)
        n125 = Unbundle By Name(w347) -> ("User Data.SubPanels"=w348:refnum<vi>[])
        n126 = Build Path(base path=w342, name or relative path="UI Setting.ini") -> (appended path=w344:path)
        n127 = call "Read UI Setting.vi"("File Path"=w344) -> ("Module Definition"=w349:T11[])  [unwired: 9 in, 1 out]
        n128 = for {
          tunnel: w349 -> [w355] mode=indexing
          tunnel: w348 -> [w354] mode=indexing
          tunnel: [w353] -> w346 mode=indexing
          n129 = call "Start Module Interface.vi"("rSubPanel"=w354, "模块定义"=w355) -> ("模块名称"=w353:string)  [unwired: 8 in, 1 out]
        }
        n130 = Bundle By Name(cluster=w347, "User Data.Interface Module List"=w346) -> (w345:T9)
        n131 = call <vilib>:"Add State(s) to Queue__JKI_lib_State_Machine.vi"("State(s) in (\"\")"=w352) -> ("States Out"=w351:string)  [unwired: 14 in]
      }
      frame "Action: Arrange SubPanels" {
        # "#CSM \"Internal State\"\nThis category is used for holding internal states"
        n132 = Unbundle By Name(w365) -> ("Core.Current VI Reference"=w358:refnum<vi>, "User Data.SubPanels"=w359:refnum<vi>[], "User Data.Interface Module List"=w356:string[])
        n133 = call "Convert API String Arguments to Data.vim"("Reference Type"=T5 {"Module Name"="", "Window Size"={"Left"=0, "Top"=0, "Right"=0, "Bottom"=0}} ("Window Size Change Arguments"), "API String"=w368) -> ("Data"=w366:T5)  [unwired: 6 in, 1 out]
        n134 = Unbundle By Name(w366) -> ("Module Name"=w364:string, "Window Size"=w361:T4)
        n135 = call "Search Unsorted 1D Array.vim"("element"=w364, "unsorted 1D array"=w356) -> ("index of element"=w363:i32)  [unwired: 9 in]
        n136 = Index Array(array=w359, index=w363) -> (element=w362:refnum<vi>)
        n137 = control-ref of="上窗格"() -> (w357:refnum<vi>)
        n138 = call "Update SubPanel Size.vi"("Window Size"=w361, "SubPanel in"=w362) -> ("error out"=w360:errorcluster)  [unwired: 9 in]
        n139 = call "Arrange SubPanels.vi"("SubPanels"=w359, "error in (no error)"=w360, "Module List"=w356, "上窗格"=w357, "VI Reference"=w358) -> ()  [unwired: 6 in, 1 out]
        n140 = call <vilib>:"Add State(s) to Queue__JKI_lib_State_Machine.vi"("State(s) in (\"\")"=w371) -> ("States Out"=w370:string)  [unwired: 14 in]
      }
      frame "Action: Launch Function" {
        # "#CSM \"Internal State\"\nThis category is used for holding internal states"
        n141 = call "Convert API String Arguments to Data.vim"("Reference Type"=T6 {"Module Name"="", "Item Name"=""} ("Item Selected Arguments"), "API String"=w381) -> ("Data"=w379:T6)  [unwired: 6 in, 1 out]
        n142 = Unbundle By Name(w379) -> ("Item Name"=w373:string, "Module Name"=w372:string)
        n143 = call "Generate Window Title.vi"("Module Name"=w372, "Item Name"=w373) -> ("Window Title"=w374:string)  [unwired: 9 in]
        n144 = case shown="\"True\"" w373 {
          tunnel: w372 -> [_ _]
          tunnel: w378 -> [w385 w392]
          tunnel: [w385 w392] -> w377
          tunnel: w376 -> [w384 w391]
          tunnel: [w384 w390] -> w375
          tunnel: w374 -> [w383 w387]
          frame "False", Default {
            n145 = One Button Dialog(message=w383) -> ()  [unwired: 1 in, 1 out]
          }
          frame "True" {
            n146 = call "Convert Data To API String Arguments.vim"("Data"=w387) -> ("API String"=w386:string)  [unwired: 7 in, 1 out]
            n147 = call <vilib>:"Build State String with Arguments__JKI_lib_State_Machine.vi"("Arguments (\"\")"=w386, "State"="Action: Register Window") -> ("State with Arguments"=w389:string)  [unwired: 4 in]
            n148 = call <vilib>:"Add State(s) to Queue__JKI_lib_State_Machine.vi"("State(s) in Front (\"\")"=w389, "State(s) in (\"\")"=w391) -> ("States Out"=w390:string)  [unwired: 13 in]
          }
        }
      }
      frame "Action: Exit Modules" {
        # "#CSM \"Category Seperator\"\nDo not put any code in this frame."
        n149 = Unbundle By Name(w394) -> ("User Data.Interface Module List"=w405:string[])
        n150 = Unbundle By Name(w394) -> ("User Data.Function Module List"=w393:set{string})
        n151 = for {
          tunnel: w393 -> [w411] mode=indexing
          n152 = call <userlib>:"CSM - Post Message.vi"("Target Module"=w411, "State"="Macro: Exit") -> ("error out"=w409:errorcluster)  [unwired: 9 in]
          n153 = call <vilib>:"Clear Errors.vi"("error in (no error)"=w409) -> ()  [unwired: 5 in, 2 out]
        }
        n154 = call <userlib>:"CSM - Unregister Broadcast.vi"("CSM Name(Empty for Broadcast Event)"=w404, "Source CSM Name (* as Default)"="*", "Trigger"="Window Size Changed", "API (\"*\" as Default)"="Action: Arrange SubPanels" ("API (If \"\", Same as Trigger)")) -> ("CSM Name (Dup)"=w403:string, "error out"=w400:errorcluster)  [unwired: 10 in]
        n155 = call <userlib>:"CSM - Unregister Broadcast.vi"("CSM Name(Empty for Broadcast Event)"=w403, "Source CSM Name (* as Default)"="*", "Trigger"="Item Selected", "API (\"*\" as Default)"="Action: Launch Function" ("API (If \"\", Same as Trigger)"), "Error In"=w400) -> ("error out"=w399:errorcluster)  [unwired: 9 in, 1 out]
        n156 = for {
          tunnel: w405 -> [w413] mode=indexing
          tunnel: w399 -> [_]
          n157 = call "Stop Module Interface.vi"("Module Name"=w413) -> ("error out"=w412:errorcluster)  [unwired: 10 in]
          n158 = call <vilib>:"Clear Errors.vi"("error in (no error)"=w412) -> ()  [unwired: 5 in, 2 out]
        }
        n159 = call <vilib>:"Add State(s) to Queue__JKI_lib_State_Machine.vi"("State(s) in (\"\")"=w408) -> ("States Out"=w407:string)  [unwired: 14 in]
      }
      frame "Action: Fix Window Width" {
        # "这里是为了防止窗口移动发生吸边的情况时变为最大化，因此在鼠标释放时强制定义窗口宽度和高度"
        # "#CSM \"Category Seperator\"\nDo not put any code in this frame."
        n160 = Unbundle By Name(w423) -> ("User Data.SubPanels"=w415:refnum<vi>[], "User Data.Interface Module List"=w414:string[], "Core.Current VI Reference"=w422:refnum<vi>)
        n161 = Unbundle By Name(w423) -> ("User Data.Window Bounds"=w426:T4)
        n162 = Unbundle By Name(w426) -> ("Right"=w424:i16, "Left"=w425:i16)
        n163 = property class="VI"(reference=w422) -> (reference out=w418:refnum<vi>, "Front Panel.WinBounds"=w421:T4)  [unwired: 1 in, 1 out]
        n164 = Subtract(x=w424, y=w425) -> (x-y=w420:i16)
        n165 = in-place {
          in-place-border: w420 -> [w432]
          n166 = in-place-cluster #1(w421) -> ("Left"=w430:i16)  [unwired: 1 out]
          n167 = Add(x=w430, y=w432) -> (x+y=w431:i16)
          n168 = in-place-cluster #1("Left"=w430, "Right"=w431) -> (w419:T4)
        }
        n169 = property class="VI"(reference=w418, "Front Panel.WinBounds"=w419) -> (reference out=w417:refnum<vi>)  [unwired: 1 in, 1 out]
        n170 = control-ref of="上窗格"() -> (w416:refnum<vi>)
        n171 = call "Arrange SubPanels.vi"("SubPanels"=w415, "Module List"=w414, "上窗格"=w416, "VI Reference"=w417) -> ()  [unwired: 7 in, 1 out]
        n172 = call <vilib>:"Add State(s) to Queue__JKI_lib_State_Machine.vi"("State(s) in (\"\")"=w429) -> ("States Out"=w428:string)  [unwired: 14 in]
      }
      frame "Action: Register Window" {
        # "#CSM \"Category Seperator\"\nDo not put any code in this frame."
        n173 = call "Convert API String Arguments to Data.vim"("Reference Type"="", "API String"=w439) -> ("Data"=w434:string)  [unwired: 6 in, 1 out]
        n174 = Unbundle By Name(w437) -> ("User Data.Function Module List"=w435:set{string})
        n175 = Insert Into Set(10:w434, 11:w435) -> (3:w433:set{string})  [unwired: 1 out]
        n176 = Bundle By Name(cluster=w437, "User Data.Function Module List"=w433) -> (w436:T9)
        n177 = call <vilib>:"Add State(s) to Queue__JKI_lib_State_Machine.vi"("State(s) in (\"\")"=w442) -> ("States Out"=w441:string)  [unwired: 14 in]
      }
      frame "Action: Unregister Window" {
        # "#CSM \"Category Seperator\"\nDo not put any code in this frame."
        n178 = Unbundle By Name(w447) -> ("User Data.Function Module List"=w446:set{string})
        n179 = call "Convert API String Arguments to Data.vim"("Reference Type"="", "API String"=w448) -> ("Data"=w445:string)  [unwired: 6 in, 1 out]
        n180 = Remove From Set(10:w445, 11:w446) -> (3:w443:set{string})  [unwired: 1 out]
        n181 = Bundle By Name(cluster=w447, "User Data.Function Module List"=w443) -> (w444:T9)
        n182 = call <vilib>:"Add State(s) to Queue__JKI_lib_State_Machine.vi"("State(s) in (\"\")"=w452) -> ("States Out"=w451:string)  [unwired: 14 in]
      }
    }
  }
